vi "XY Graph NXG with TipStrip.vi"() -> ()   [LabVIEW 2021, in "XY Graph Add-Ons.lvlib"]
uses:
  XY Graph Add-Ons.lvlib
  XY Graph Plot Data.ctl
  XY Graph Refnum.ctl
panel:
  out "XY Graph TipStrip":string
  out "XY Graph":cluster{"X Array":dbl[], "Y Array":dbl[]}[](graph)
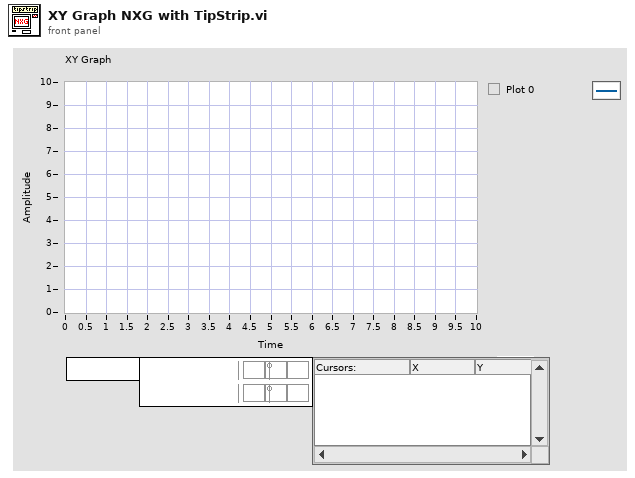
[diagram p1: front panel]
types:
  T1 = cluster{"XY Graph TipStrip":refnum<event-registration>}
  T2 = typedef "XY Graph Add-Ons.lvlib/XY Graph Plot Data.ctl" = cluster{"X Array":dbl[], "Y Array":dbl[]}
  T3 = typedef "LVPoint32TypeDef.ctl" = cluster{"Horizontal":i32, "Vertical":i32}
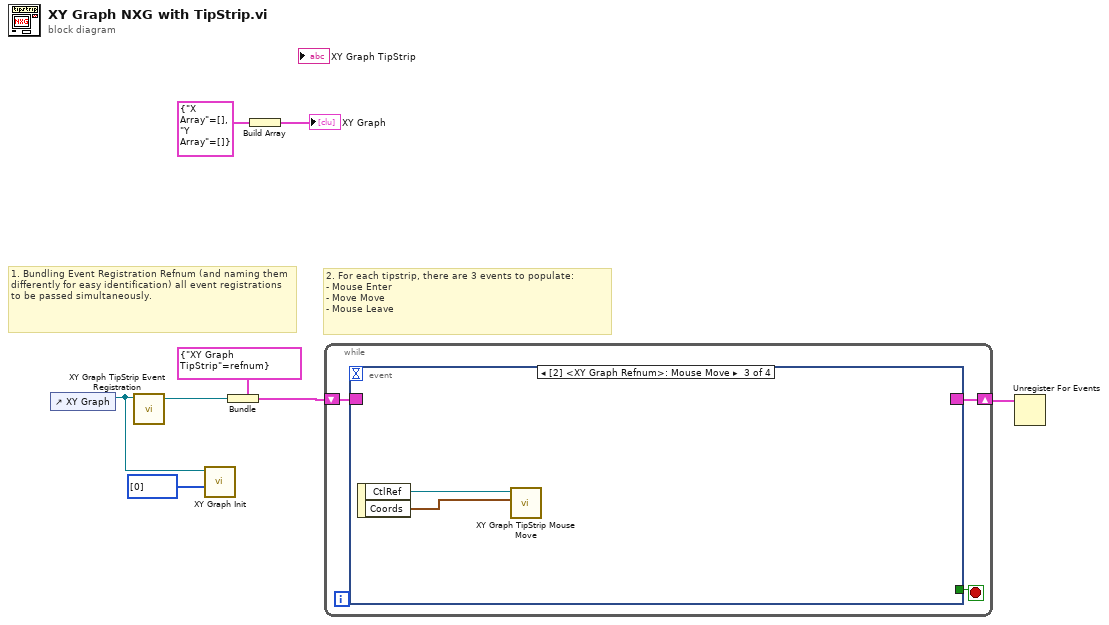
[diagram p0: block diagram]
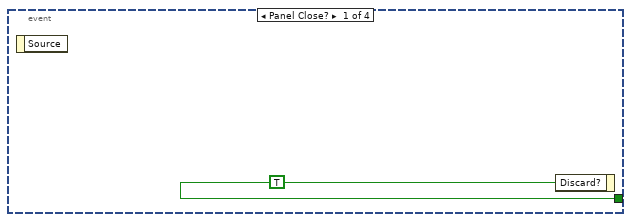
[diagram p2: hidden frame]
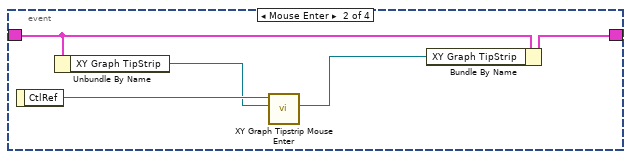
[diagram p3: hidden frame]
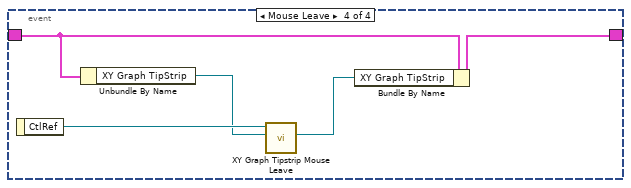
[diagram p4: hidden frame]
diagram:
  # "2. For each tipstrip, there are 3 events to populate:\n- Mouse Enter\n- Move Move\n- Mouse Leave"
  # "1. Bundling Event Registration Refnum (and naming them differently for easy identification) all event registrations to be passed simultaneously."
  n1 = control-ref of="XY Graph"() -> (w1:refnum<vi>)
  n2 = call "XY Graph TipStrip Event Registration.vi"("XY Graph Refnum"=w1) -> ("Event Registration Refnum"=w6:refnum<event-registration>)  [unwired: 8 in, 2 out]
  n3 = call "XY Graph Init.vi"("Plots to Skip (none)"=i32[] [0], "XYGraph in"=w1) -> ()  [unwired: 9 in, 1 out]
  n4 = Bundle(cluster=T1 {"XY Graph TipStrip"=refnum} ("Event Registration Refnums"), "XY Graph TipStrip"=w6) -> (w4:T1)
  n5 = Build Array(T2 {"X Array"=[], "Y Array"=[]} ("Plot")) -> (→"XY Graph":T2[])
  n6 = while {
    shift-right: [w9] -> w5
    shift-left: w4 -> [w11]
    stop <- w10 stop-if-true
    n7 = event shown="[2] <XY Graph Refnum>: Mouse Move" {
      selector: w11 -> [_ w15 _ w21]
      dyn-events: [_ w17 _ w20] -> w9
      timeout: _ -> [_ _ _ _]
      tunnel: [w12 _ _ _] -> w10
      event Panel Close? {
        w12 = TRUE ("Discard?")
        n8 = event-data() -> ()  [unwired: 1 in, 1 out]
        n9 = event-data("Discard?"=w12) -> ()  [unwired: 1 in, 1 out]
      }
      event Mouse Enter {
        n10 = event-data() -> ("CtlRef"=w16:refnum<vi>)  [unwired: 1 in]
        n11 = Unbundle By Name(w15) -> ("XY Graph TipStrip"=w14:refnum<event-registration>)
        n12 = call "XY Graph Tipstrip Mouse Enter.vi"("Event Registration Refnum"=w14, "XY Graph Refnum"=w16) -> ("Event Registration Refnum"=w13:refnum<event-registration>)  [unwired: 8 in, 1 out]
        n13 = Bundle By Name(cluster=w15, "XY Graph TipStrip"=w13) -> (w17:T1)
      }
      event Mouse Move {
        n14 = event-data() -> ("CtlRef"=w19:refnum<vi>, "Coords"=w18:T3)  [unwired: 1 in]
        n15 = call "XY Graph TipStrip Mouse Move.vi"("Coords"=w18, "XY Graph Refnum"=w19) -> ()  [unwired: 7 in, 3 out]
      }
      event Mouse Leave {
        n16 = event-data() -> ("CtlRef"=w24:refnum<vi>)  [unwired: 1 in]
        n17 = Unbundle By Name(w21) -> ("XY Graph TipStrip"=w23:refnum<event-registration>)
        n18 = call "XY Graph Tipstrip Mouse Leave.vi"("Event Registration Refnum"=w23, "XY Graph Refnum"=w24) -> ("Event Registration Refnum"=w22:refnum<event-registration>)  [unwired: 8 in, 1 out]
        n19 = Bundle By Name(cluster=w21, "XY Graph TipStrip"=w22) -> (w20:T1)
      }
    }
  }
  n20 = Unregister For Events(event registration refnum=w5) -> ()  [unwired: 1 in, 1 out]
